vi "Add Child UID To Parent List.vi"(0 "Base Tree in":refnum<class "Base Tree.lvclass">, 1 "UID":string, 2 "ParentUID":string, 3 "error in (no error)":errorcluster) -> (7 "Base Tree out":refnum<class "Base Tree.lvclass">, 10 "error out":errorcluster)   [LabVIEW 2017, in "Browser Core.lvlib" / "Base Tree.lvclass"]
doc: "Add UID to the list of Children of the Parent Class"
uses:
  Base Tree.lvclass
  Base Tree.lvclass/Base Tree.ctl
  Node Classes/Generic Node/Generic Node.lvclass
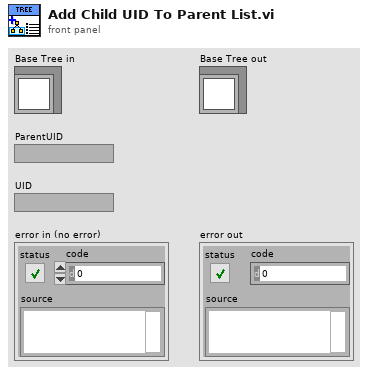
[diagram p1: front panel]
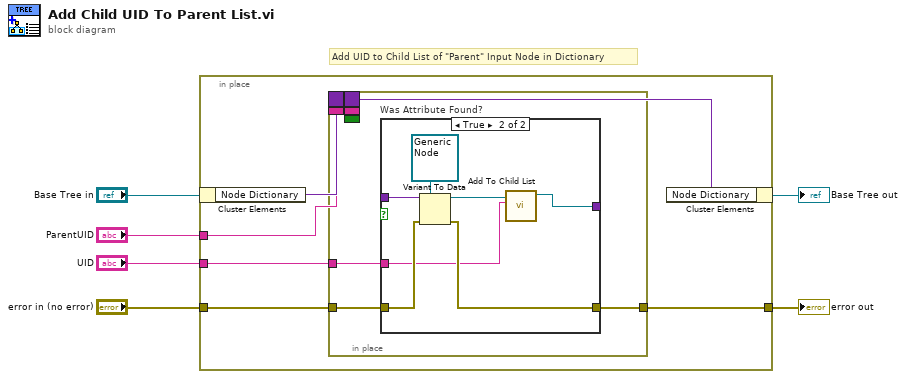
[diagram p0: block diagram]
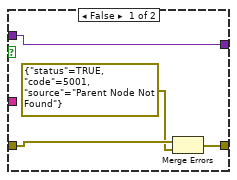
[diagram p2: hidden frame]
diagram:
  # "Add UID to Child List of \"Parent\" Input Node in Dictionary"
  n1 = in-place {
    in-place-border: "error in (no error)" -> [w10]
    in-place-border: "UID" -> [w7]
    in-place-border: "ParentUID" -> [w9]
    in-place-border: [w8] -> w3
    n2 = in-place-cluster #1("Base Tree in") -> ("Node Dictionary"=w12:variant)
    n3 = in-place {
      border: w12 -> [_]
      border: w9 -> [_]
      border: [_] -> w11
      border: _ -> [_]
      border: _ -> [_]
      in-place-border: w10 -> [w16]
      in-place-border: [w14] -> w8
      in-place-border: w7 -> [w13]
      n4 = case "Was Attribute Found?" shown="True" w18 {
        tunnel: w17 -> [w22 w29]
        tunnel: w16 -> [w20 w26]
        tunnel: [w22 w23] -> w15
        tunnel: [w21 w25] -> w14
        tunnel: w13 -> [_ w24]
        frame False {
          n5 = Merge Errors(w20, errorcluster {"status"=TRUE, "code"=5001, "source"="Parent Node Not Found"} ("error in (no error)")) -> (w21:errorcluster)
        }
        frame True {
          n6 = Variant To Data(error in=w26, type=refnum<class "Generic Node.lvclass"> refnum ("New Node"), Variant=w29) -> (data=w27:refnum<class "Generic Node.lvclass">, error out=w25:errorcluster)
          n7 = call-dynamic "Add To Child List.vi"("Child ID"=w24, "Generic Node in"=w27) -> ("Generic Node out"=w23:refnum<class "Generic Node.lvclass">)  [unwired: 9 in]
        }
      }
    }
    n8 = in-place-cluster #1("Node Dictionary"=w11) -> (→"Base Tree out":refnum<class "Base Tree.lvclass">)
  }
  "error out" <- w3
